vi "initCommandList.vi"() -> ()   [LabVIEW 2010]
uses:
  VarableID.ctl
  GlobalCostants.vi
panel:
  in  "CommandCodeList":cluster{"CommandCode":string, "VarableID":T1}[](array[cluster])=[{"CommandCode"="68####68110402020100", "VarableID"=enum."current"}, {"CommandCode"="68####68110433343435", "VarableID"=enum."voltage"}, {"CommandCode"="68####68110402050100", "VarableID"=enum."power"}, {"CommandCode"="68####68110402060100", "VarableID"=enum."PF"}]
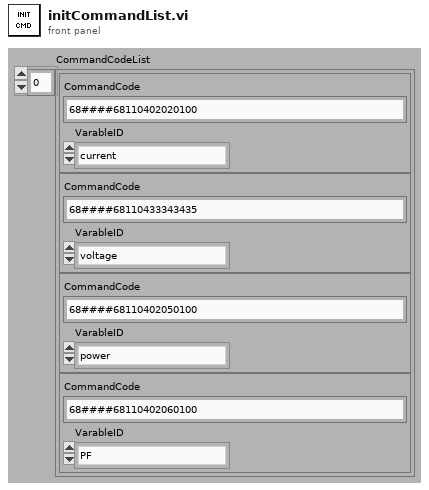
[diagram p1: front panel]
types:
  T1 = typedef "VarableID.ctl" = enum16{"current", "voltage", "power", "PF"}
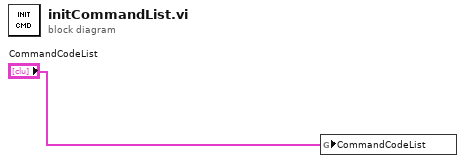
[diagram p0: block diagram]
diagram:
  n1 = global write "GlobalCostants.vi" "CommandCodeList"("CommandCodeList") -> ()
